vi "Enable Output.vi"(8 "error in (no error)":errorcluster, 10 "Enable Output (F: Disabled)":bool, 11 "VISA resource name":refnum<visa-resource-name>) -> (0 "error out":errorcluster, 3 "VISA resource name out":refnum<visa-resource-name>)   [LabVIEW 2022 SP3, in "BK Precision 9103.lvlib"]
doc: "Enables or disables the output."
uses:
  <instrlib>/BK Precision 9103/BK Precision 9103.lvlib
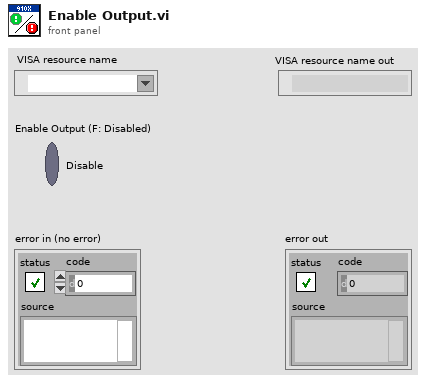
[diagram p1: front panel]
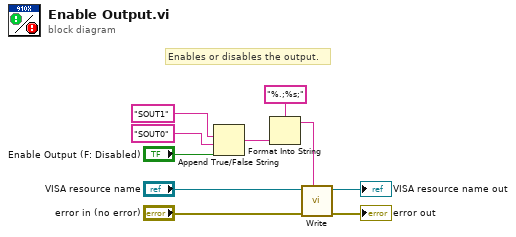
[diagram p0: block diagram]
diagram:
  # "Enables or disables the output."
  n1 = Append True/False String(1:"Enable Output (F: Disabled)", 2:"SOUT0", 3:"SOUT1") -> (0:w6:string)  [unwired: 1 in]
  n2 = Format Into String(format string="%.;%s;", w6) -> (resulting string=w5:string)  [unwired: 2 in, 1 out]
  n3 = call <instrlib>:"Write.vi"("Input String"=w5, "error in (no error)"="error in (no error)", "VISA resource name"="VISA resource name") -> ("error out"=→"error out":errorcluster, "VISA resource name out"=→"VISA resource name out":refnum<visa-resource-name>)  [unwired: 6 in, 1 out]
